vi "ChapR cRIO Translater.vi"(6 "Position":u8=49, 7 "CMD":u8, 8 "Alliance":u8=66, 9 "Digtl In":u8, 10 "ChapR Data":string, 11 "TeamNo":u16) -> (2 "Network Data":string)   [LabVIEW 2013]
uses:
  ChapR Packet.ctl
  Driver Station Packet.ctl
panel:
  out "value":T1
  in  "Network Packet 2":T1
  in  "Network Packet":T1
  in  "ChapR Packet":T2
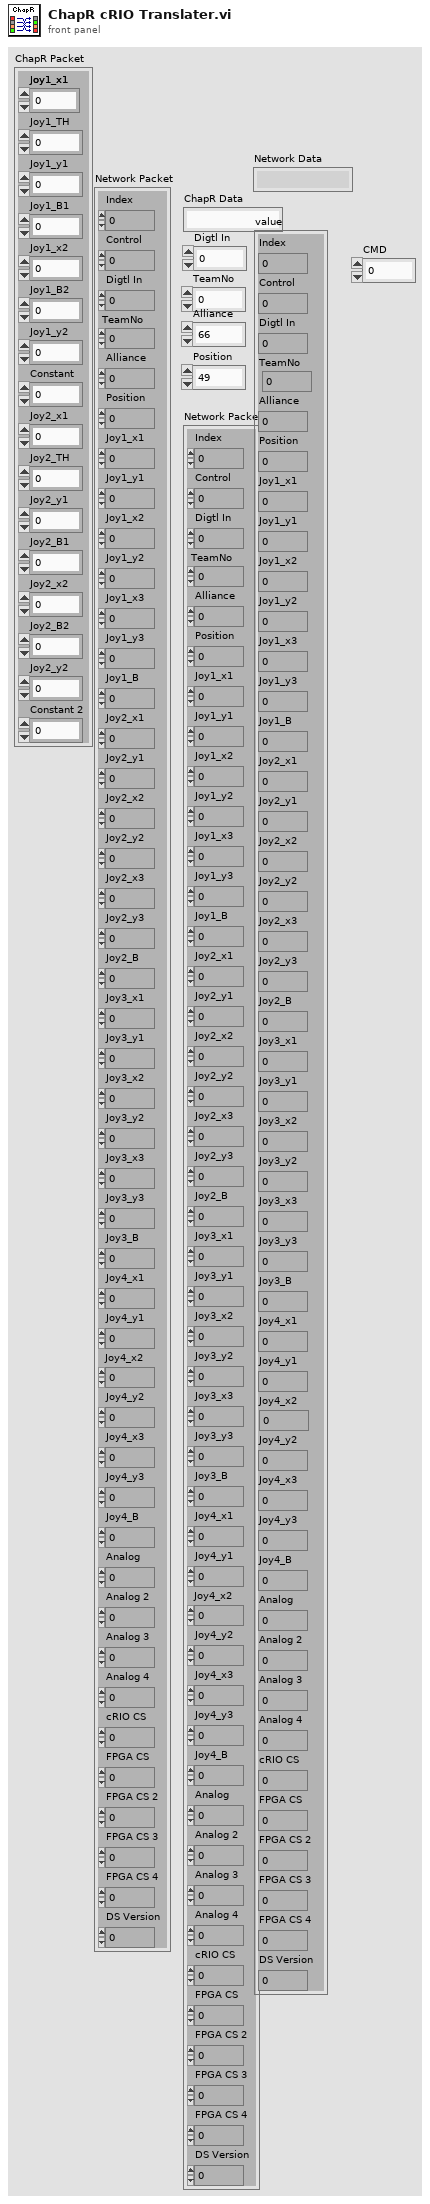
[diagram p1: front panel]
types:
  T1 = typedef "Driver Station Packet.ctl" = cluster{"Index":u16, "Control":u8, "Digtl In":u8, "TeamNo":u16, "Alliance":u8, "Position":u8, "Joy1_x1":i8, "Joy1_y1":i8, "Joy1_x2":i8, "Joy1_y2":i8, "Joy1_x3":i8, "Joy1_y3":i8, "Joy1_B":u16, "Joy2_x1":i8, "Joy2_y1":i8, "Joy2_x2":i8, "Joy2_y2":i8, "Joy2_x3":i8, "Joy2_y3":i8, "Joy2_B":u16, "Joy3_x1":i8, "Joy3_y1":i8, "Joy3_x2":i8, "Joy3_y2":i8, "Joy3_x3":i8, "Joy3_y3":i8, "Joy3_B":u16, "Joy4_x1":i8, "Joy4_y1":i8, "Joy4_x2":i8, "Joy4_y2":i8, "Joy4_x3 ":i8, "Joy4_y3":i8, "Joy4_B":u16, "Analog":u16, "Analog 2":u16, "Analog 3":u16, "Analog 4":u16, "cRIO CS":u64, "FPGA CS":u32, "FPGA CS 2":u32, "FPGA CS 3":u32, "FPGA CS 4":u32, "DS Version":u64}
  T2 = typedef "ChapR Packet.ctl" = cluster{"Joy1_x1":i8, "Joy1_TH":u8, "Joy1_y1":i8, "Joy1_B1":u8, "Joy1_x2":i8, "Joy1_B2":u8, "Joy1_y2":i8, "Constant":u8, "Joy2_x1":i8, "Joy2_TH":u8, "Joy2_y1":i8, "Joy2_B1":u8, "Joy2_x2":i8, "Joy2_B2":u8, "Joy2_y2":i8, "Constant 2":u8}
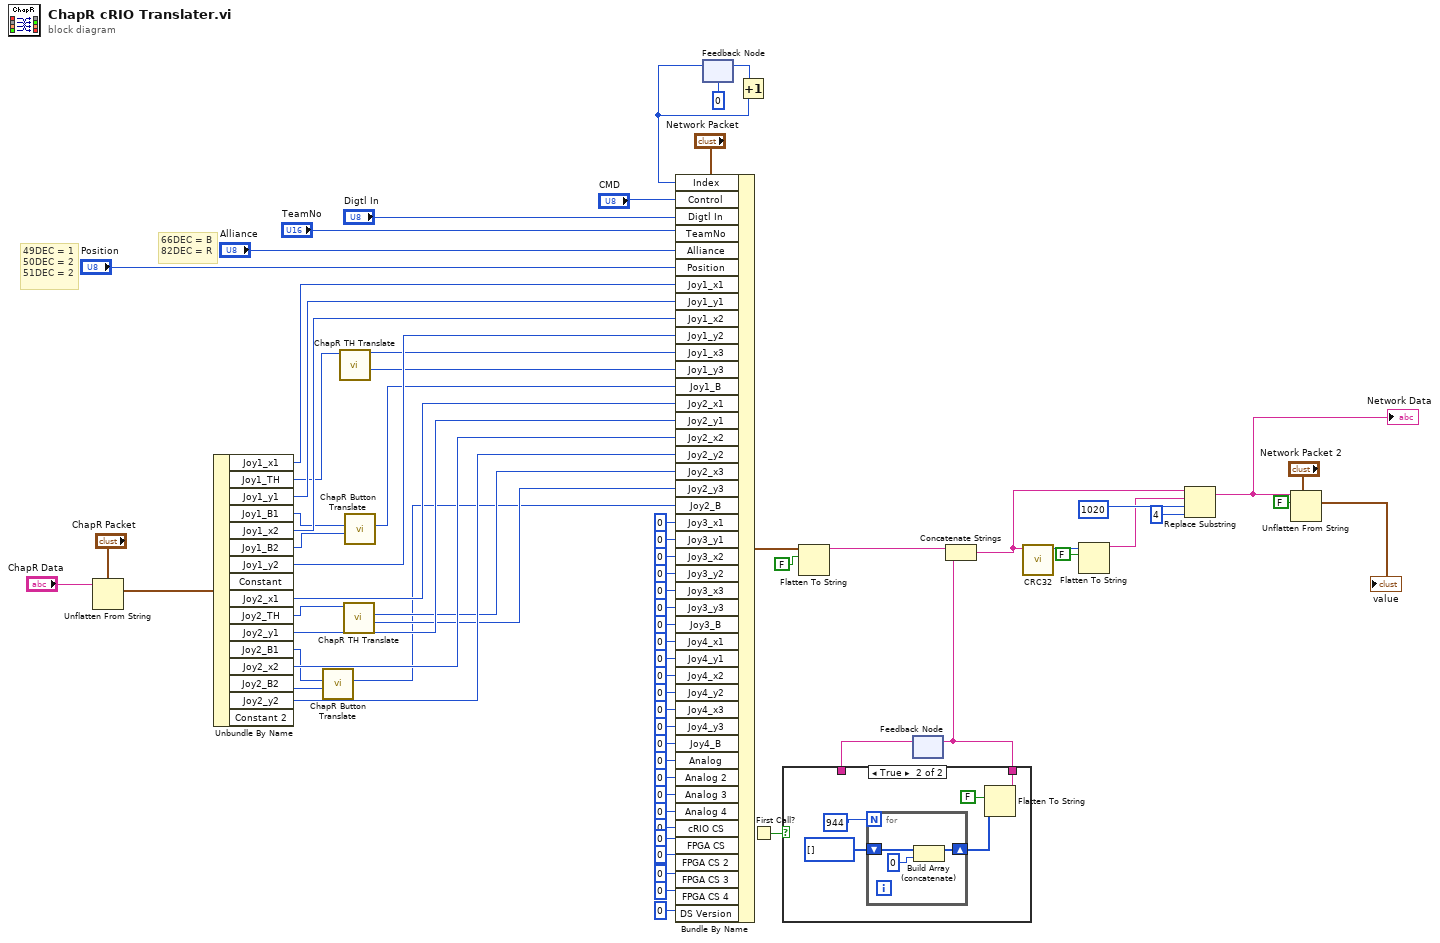
[diagram p0: block diagram]
diagram:
  # "49DEC = 1\n50DEC = 2\n51DEC = 2"
  # "66DEC = B\n82DEC = R"
  n1 = Unflatten From String(type="ChapR Packet", binary string="ChapR Data") -> (value=w62:T2)  [unwired: 3 in, 2 out]
  n2 = Unbundle By Name(w62) -> ("Joy1_x1"=w71:i8, "Joy1_TH"=w59:u8, "Joy1_y1"=w70:i8, "Joy1_B1"=w53:u8, "Joy1_x2"=w68:i8, "Joy1_B2"=w52:u8, "Joy1_y2"=w67:i8, "Joy2_x1"=w66:i8, "Joy2_TH"=w56:u8, "Joy2_y1"=w69:i8, "Joy2_B1"=w50:u8, "Joy2_x2"=w65:i8, "Joy2_B2"=w49:u8, "Joy2_y2"=w64:i8)  [unwired: 2 out]
  n3 = call "ChapR Button Translate.vi"("B2"=w49, "B1"=w50) -> ("B"=w24:u16)  [unwired: 9 in]
  n4 = call "ChapR TH Translate.vi"("Tophat Value"=w59) -> ("Y"=w57:i8, "X"=w58:i8)  [unwired: 9 in]
  n5 = call "ChapR TH Translate.vi"("Tophat Value"=w56) -> ("Y"=w55:i8, "X"=w54:i8)  [unwired: 9 in]
  n6 = call "ChapR Button Translate.vi"("B2"=w52, "B1"=w53) -> ("B"=w51:u16)  [unwired: 9 in]
  n7 = feedback #1(u16 0) -> (w22:u16)
  n8 = Bundle By Name(cluster="Network Packet", "Index"=w22, "Control"="CMD", "Digtl In"="Digtl In", "TeamNo"="TeamNo", "Alliance"="Alliance", "Position"="Position", "Joy1_x1"=w71, "Joy1_y1"=w70, "Joy1_x2"=w68, "Joy1_y2"=w67, "Joy1_x3"=w58, "Joy1_y3"=w57, "Joy1_B"=w51, "Joy2_x1"=w66, "Joy2_y1"=w69, "Joy2_x2"=w65, "Joy2_y2"=w64, "Joy2_x3"=w54, "Joy2_y3"=w55, "Joy2_B"=w24, "Joy3_x1"=i8 0, "Joy3_y1"=i8 0, "Joy3_x2"=i8 0, "Joy3_y2"=i8 0, "Joy3_x3"=i8 0, "Joy3_y3"=i8 0, "Joy3_B"=u16 0, "Joy4_x1"=i8 0, "Joy4_y1"=i8 0, "Joy4_x2"=i8 0, "Joy4_y2"=i8 0, "Joy4_x3"=i8 0, "Joy4_y3"=i8 0, "Joy4_B"=u16 0, "Analog"=u16 0, "Analog 2"=u16 0, "Analog 3"=u16 0, "Analog 4"=u16 0, "cRIO CS"=u64 0, "FPGA CS"=u32 0, "FPGA CS 2"=u32 0, "FPGA CS 3"=u32 0, "FPGA CS 4"=u32 0, "DS Version"=u64 0) -> (w61:T1)
  n9 = Increment(x=w22) -> (x+1=w21:u16)
  n10 = feedback-in #1(w21) -> ()
  n11 = First Call?() -> (First Call?: T/F=w7:bool)
  n12 = Flatten To String(anything=w61, prepend array or string size? (T)=FALSE) -> (data string=w4:string)  [unwired: 2 in, 2 out]
  n13 = feedback #2() -> (w6:string)  [unwired: 1 in]
  n14 = case shown="True" w7 {
    tunnel: [w73 w75] -> w3
    tunnel: w6 -> [w73 _]
    frame False {
    }
    frame True {
      n15 = for {
        N: 944 -> [_]
        shift-right: [w79] -> w76
        shift-left: u8[] [] -> [w81]
        n16 = Build Array (concatenate)(w81, u8 0) -> (w79:u8[])
      }
      n17 = Flatten To String(anything=w76, prepend array or string size? (T)=FALSE) -> (data string=w75:string)  [unwired: 2 in, 2 out]
    }
  }
  n18 = feedback-in #2(w3) -> ()
  n19 = Concatenate Strings(w4, w3) -> (w5:string)
  n20 = call "CRC32.vi"("Data"=w5) -> ("CRC32Value"=w14:u32)  [unwired: 10 in]
  n21 = Flatten To String(anything=w14, prepend array or string size? (T)=FALSE) -> (data string=w13:string)  [unwired: 2 in, 2 out]
  n22 = Replace Substring(2:4 ("length (len. of substring)"), 3:1020 ("offset (0)"), 4:w13, 5:w5) -> (1:w2:string)  [unwired: 1 out]
  "Network Data" <- w2
  n23 = Unflatten From String(type="Network Packet 2", binary string=w2, data includes array or string size? (T)=FALSE) -> (value=→"value":T1)  [unwired: 2 in, 2 out]
